vi "Execute GC EX Vacuum Test.vi"(8 "error in":errorcluster, 9 "Test Results":T1, 10 "Gas":T3, 11 "GC EX Configuration":T4) -> (0 "error out":errorcluster, 1 "Test Results Out":T1, 2 "Gas Out":T3 caption="Gas", 3 "GC Configuration Out":T4)   [LabVIEW 2015]
uses:
  Controls/Test Information.ctl
  Controls/Vacuum Test.ctl
  Controls/Test Timing.ctl
  Controls/Vaccum Thresholds.ctl
  Controls/Helium Test.ctl
  Controls/Helium Thresholds.ctl
  CAN Communication/Gas/Typedefs/Session Handle.ctl
  CAN Communication/Gas/Gas.lvclass
  Controls/Test Results.ctl
  Controls/Step Result.ctl
  User Interface/UI Handler/UI Handler.lvclass
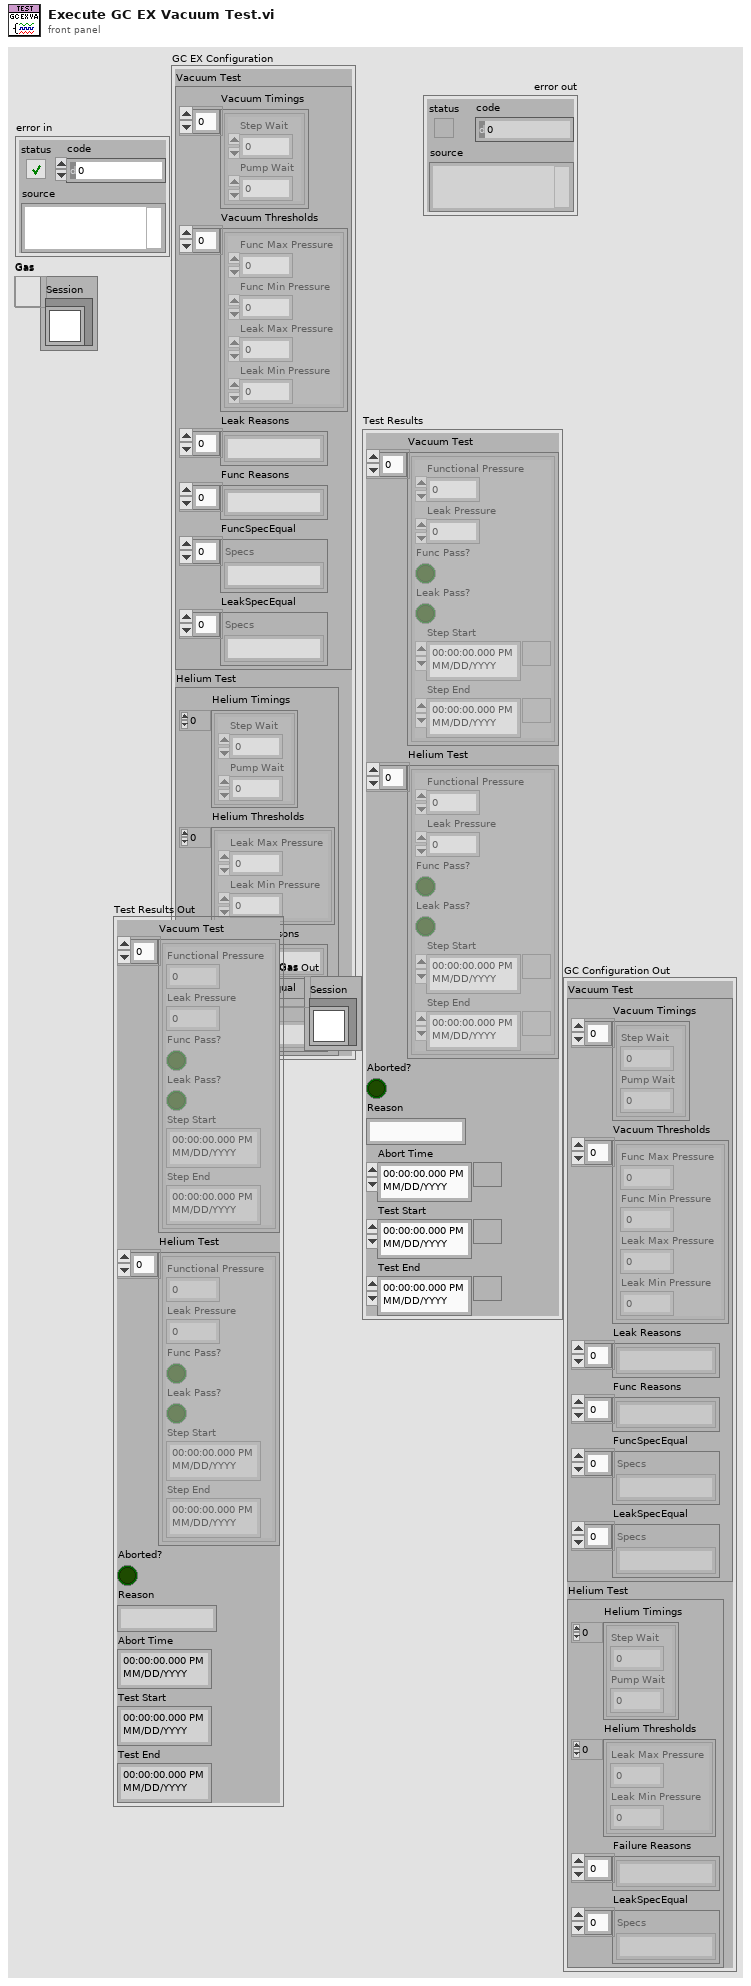
[diagram p1: front panel]
types:
  T1 = typedef "Test Results.ctl" = cluster{"Vacuum Test":T2[], "Helium Test":T2[], "Aborted?":bool, "Reason":string, "Abort Time":timestamp, "Test Start":timestamp, "Test End":timestamp}
  T2 = typedef "Step Result.ctl" = cluster{"Functional Pressure":dbl, "Leak Pressure":dbl, "Func Pass?":bool, "Leak Pass?":bool, "Step Start":timestamp, "Step End":timestamp}
  T3 = typedef "Gas.lvclass/Session Handle.ctl" = refnum<data-value>
  T4 = typedef "Test Information.ctl" = cluster{"Vacuum Test":T5, "Helium Test":T8}
  T5 = typedef "Vacuum Test.ctl" = cluster{"Vacuum Timings":T6[], "Vacuum Thresholds":T7[], "Leak Reasons":string[], "Func Reasons":string[], "FuncSpecEqual":string[], "LeakSpecEqual":string[]}
  T6 = typedef "Test Timing.ctl" = cluster{"Step Wait":dbl, "Pump Wait":dbl}
  T7 = typedef "Vaccum Thresholds.ctl" = cluster{"Func Max Pressure":dbl, "Func Min Pressure":dbl, "Leak Max Pressure":dbl, "Leak Min Pressure":dbl}
  T8 = typedef "Helium Test.ctl" = cluster{"Helium Timings":T6[], "Helium Thresholds":T9[], "Failure Reasons":string[], "LeakSpecEqual":string[]}
  T9 = typedef "Helium Thresholds.ctl" = cluster{"Leak Max Pressure":dbl, "Leak Min Pressure":dbl}
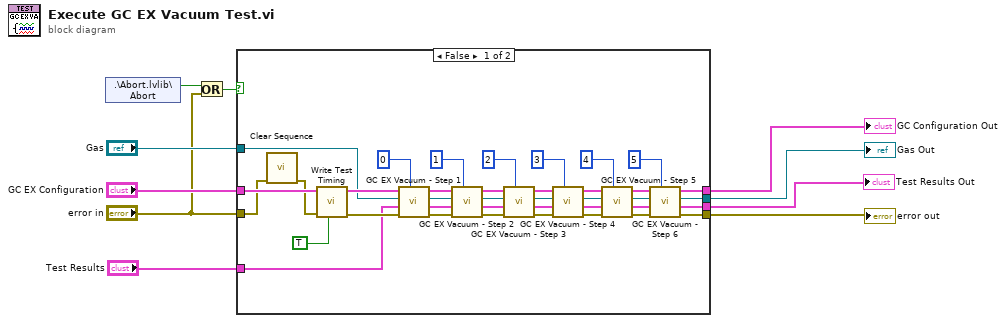
[diagram p0: block diagram]
diagram:
  n1 = shared-variable ".\\Abort.lvlib\\Abort"() -> (w3:bool)  [unwired: 1 in, 1 out]
  n2 = Or(x=w3, y="error in") -> (x .or. y?=w1:bool)
  n3 = case shown="False" w1 {
    tunnel: "error in" -> [w18 w49]
    tunnel: "GC EX Configuration" -> [w45 w51]
    tunnel: "Gas" -> [w44 w50]
    tunnel: "Test Results" -> [w43 w48]
    tunnel: [w12 w49] -> w7
    tunnel: [w15 w51] -> w6
    tunnel: [w14 w50] -> w5
    tunnel: [w13 w48] -> w4
    frame False {
      n4 = call "Clear Sequence.vi"("error in (no error)"=w18) -> ("error out"=w17:errorcluster)  [unwired: 10 in]
      n5 = call "Write Test Timing.vi"("Vacuum?"=TRUE, "error in (no error)"=w17, "Test Information"=w45) -> ("error out"=w46:errorcluster)  [unwired: 8 in]
      n6 = call "GC EX Vacuum - Step 1.vi"("Step"=0, "error in"=w46, "Test Results In"=w43, "Gas"=w44, "GC Configuration"=w45) -> ("error out"=w39:errorcluster, "Test Results Out"=w40:T1, "Gas Out"=w41:T3, "GC Configuration Out"=w42:T4)  [unwired: 3 in]
      n7 = call "GC EX Vacuum - Step 2.vi"("Step"=1, "error in"=w39, "Test Results In"=w40, "Gas"=w41, "GC Configuration"=w42) -> ("error out"=w37:errorcluster, "Test Results Out"=w11:T1, "Gas Out"=w35:T3, "GC Configuration Out"=w36:T4)  [unwired: 3 in]
      n8 = call "GC EX Vacuum - Step 3.vi"("Step"=2, "error in"=w37, "Test Results In"=w11, "Gas"=w35, "GC Configuration"=w36) -> ("error out"=w33:errorcluster, "Test Results Out"=w30:T1, "Gas Out"=w31:T3, "GC Configuration Out"=w32:T4)  [unwired: 3 in]
      n9 = call "GC EX Vacuum - Step 4.vi"("Step"=3, "error in"=w33, "Test Results In"=w30, "Gas"=w31, "GC Configuration"=w32) -> ("error out"=w27:errorcluster, "Test Results Out"=w25:T1, "Gas Out"=w26:T3, "GC Configuration Out"=w28:T4)  [unwired: 3 in]
      n10 = call "GC EX Vacuum - Step 5.vi"("Step"=4, "error in"=w27, "Test Results In"=w25, "Gas"=w26, "GC Configuration"=w28) -> ("error out"=w23:errorcluster, "Test Results Out"=w20:T1, "Gas Out"=w21:T3, "GC Configuration Out"=w22:T4)  [unwired: 3 in]
      n11 = call "GC EX Vacuum - Step 6.vi"("Step"=5, "error in"=w23, "Test Results In"=w20, "Gas"=w21, "GC Configuration"=w22) -> ("error out"=w12:errorcluster, "Test Results Out"=w13:T1, "Gas Out"=w14:T3, "GC Configuration Out"=w15:T4)  [unwired: 3 in]
    }
    frame True {
    }
  }
  "error out" <- w7
  "GC Configuration Out" <- w6
  "Gas Out" <- w5
  "Test Results Out" <- w4
